vi "Verify and Check-in.vi"(0 "Hotel Management Tool Model in":refnum<class "Hotel Management Tool Model.lvclass">, 5 "Rooms Manager GUID":string, 7 "Room No":string, 9 "Guest Contact Number In":string caption="Guest Contact Number", 11 "error in (no error)":errorcluster, 12 "Primary Guest Name":string, 13 "Adults":u32, 14 "Children":u32) -> (4 "Hotel Management Tool Model out":refnum<class "Hotel Management Tool Model.lvclass">, 15 "error out":errorcluster)   [LabVIEW 2023, in "Hotel Management Tool Model.lvlib" / "Hotel Management Tool Model.lvclass"]
uses:
  Hotel Management Tool Model.lvclass
  Hotel Management Tool Model.lvclass/Hotel Management Tool Model.ctl
  Central Data Manager/Central Data Manager Messages/Verify and Check-In Msg/Verify and Check-In Msg.lvclass
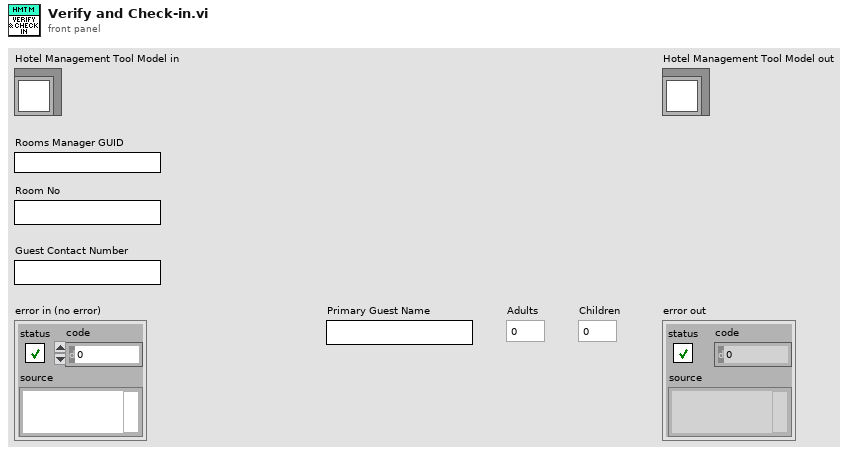
[diagram p1: front panel]
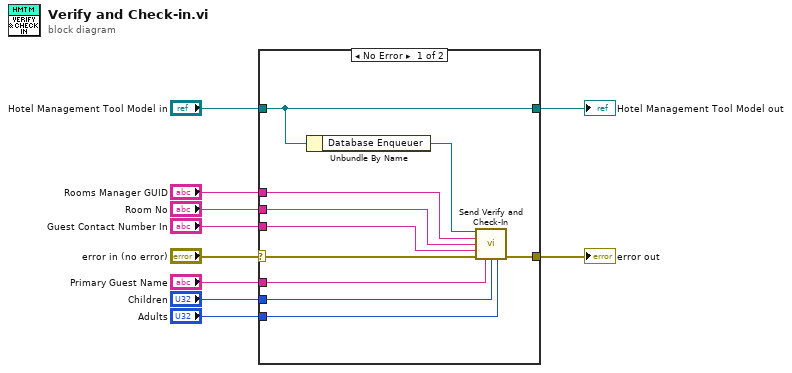
[diagram p0: block diagram]
diagram:
  n1 = case shown="No Error" "error in (no error)" {
    selector: "error in (no error)" -> [w18 w22]
    tunnel: [w19 w22] -> w9
    tunnel: [w20 w21] -> w8
    tunnel: "Hotel Management Tool Model in" -> [w20 w21]
    tunnel: "Room No" -> [w12 _]
    tunnel: "Guest Contact Number In" -> [w11 _]
    tunnel: "Rooms Manager GUID" -> [w13 _]
    tunnel: "Primary Guest Name" -> [w16 _]
    tunnel: "Children" -> [w15 _]
    tunnel: "Adults" -> [w14 _]
    frame No Error {
      n2 = Unbundle By Name(w20) -> ("Database Enqueuer"=w17:refnum<class "Message Enqueuer.lvclass">)
      n3 = call "Send Verify and Check-In.vi"("Message Enqueuer"=w17, "Rooms Manager GUID"=w13, "Room No"=w12, "Guest Contact Number In"=w11, "error in (no error)"=w18, "Primary Guest Name"=w16, "Adults"=w15, "Children"=w14) -> ("error out"=w19:errorcluster)  [unwired: 6 in, 1 out]
    }
    frame Error {
    }
  }
  "error out" <- w9
  "Hotel Management Tool Model out" <- w8
